vi "Main.Resize.vi"(10 "Sub Panel":refnum<vi>, 11 "VI in":refnum<vi>) -> ()   [LabVIEW 2019]
uses:
  <vilib>/Utility/miscctls.llb/LVPointTypeDef.ctl
  Users/Nicole/Downloads/a/ims-desktop/Variaveis/WindowAppearance.vi
  Users/Nicole/Downloads/a/ims-desktop/Variaveis/Config.vi
  Users/Nicole/Downloads/a/ims-desktop/Variaveis/Cnc.vi
  Users/Nicole/Downloads/a/ims-desktop/Variaveis/Checklist.vi
  Users/Nicole/Downloads/a/ims-desktop/Variaveis/NetworkShortcutLink.vi
  Users/Nicole/Downloads/a/ims-desktop/Variaveis/ProductionOrderConfiguration.vi
  Users/Nicole/Downloads/a/ims-desktop/Variaveis/CharacteristicVisualization.vi
  Users/Nicole/Downloads/a/ims-desktop/Variaveis/AnalogDigitalIOs.vi
panel:
  out "SFMVisible":bool
  out "ENSVisible":bool
  out "Position":dbl
  out "SubPnlTop":i32
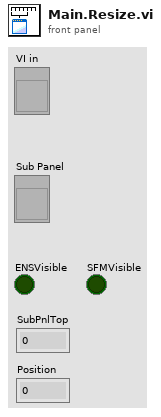
[diagram p1: front panel]
types:
  T1 = enum32{"Invalid", "Standard", "Closed", "Hidden", "Minimized", "Maximized"}
  T2 = typedef "LVPointTypeDef.ctl" = cluster{"Horizontal":i16, "Vertical":i16}
  T3 = typedef "LVAllMonitorsDisplayTypeDef.ctl" = cluster{"Bounds":cluster{"Left":i16, "Top":i16, "Right":i16, "Bottom":i16}, "Depth":i16}[]
  T4 = cluster{"Bounds":cluster{"Left":i16, "Top":i16, "Right":i16, "Bottom":i16}, "Depth":i16}
  T5 = cluster{"Left":i16, "Top":i16, "Right":i16, "Bottom":i16}
  T6 = cluster{"EnsPanelCode":i32, "GcfWorkcenterId":i32, "MeasurementType":i32, "SmartkattTemporaryFolder":path, "SmartkattReelFolder":path, "SmartkattConfiguration":string[][], "PrintReelLabel":bool, "Wire.TimeToCheckStatus":i32, "Wire.SegmentLength":i32, "EnablePopupAfterReelCut":bool}
  T7 = typedef "Msm.Checklist.ctl" = cluster{"checklistId":string, "plantId":i32, "departmentId":i32, "title":string, "version":i32, "createDate":timestamp, "userCreate":string, "language":string, "enabled":bool, "lists":cluster{"sequence":i32, "title":string, "description":string, "items":cluster{"sequence":i32, "title":string, "description":string, "type":enum16{"quantitative", "qualitative", "descriptive", "formula", "ensFindValue", "ensCharacteristic"}, "linearPosition":dbl, "angularPosition":dbl, "nominalValue":dbl, "minimumValue":dbl, "maximumValue":dbl, "unitOfMeasurement":string, "formula":string, "characteristic":string, "equipmentType":i32, "allowToleranceEdit":bool, "equipmentConfiguration":string}[]}[]}
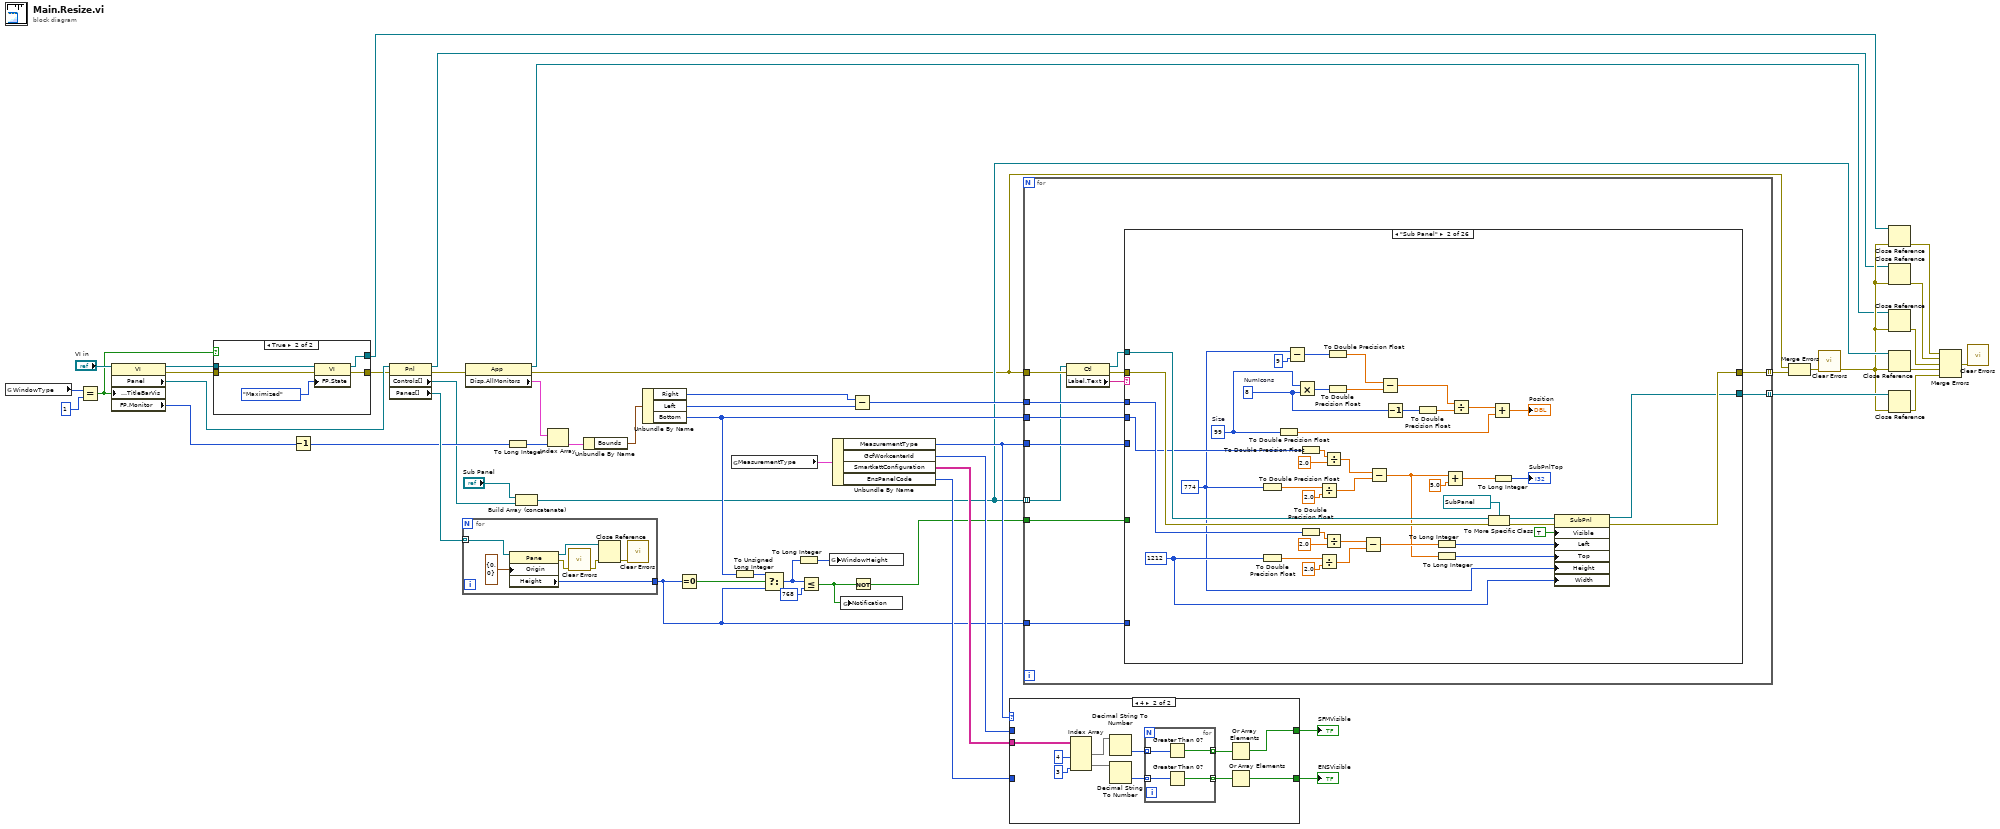
[diagram p0: block diagram]
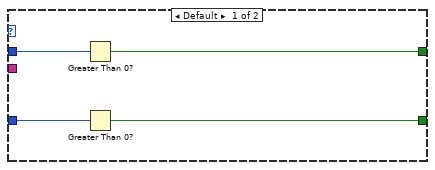
[diagram p3: hidden frame]
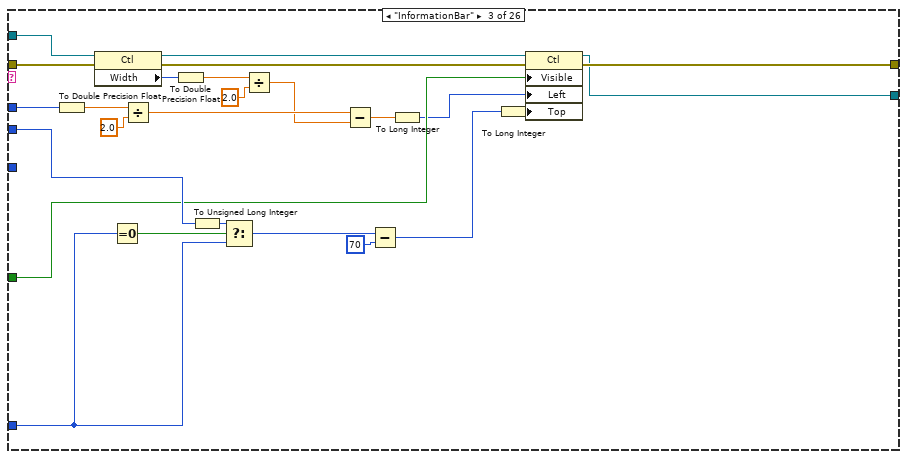
[diagram p5: hidden frame]
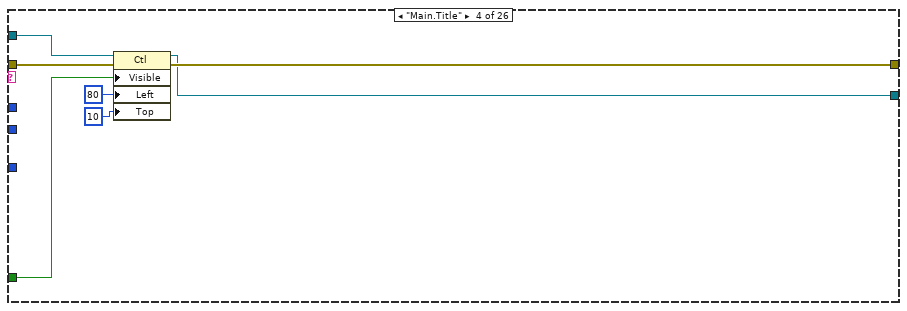
[diagram p6: hidden frame]
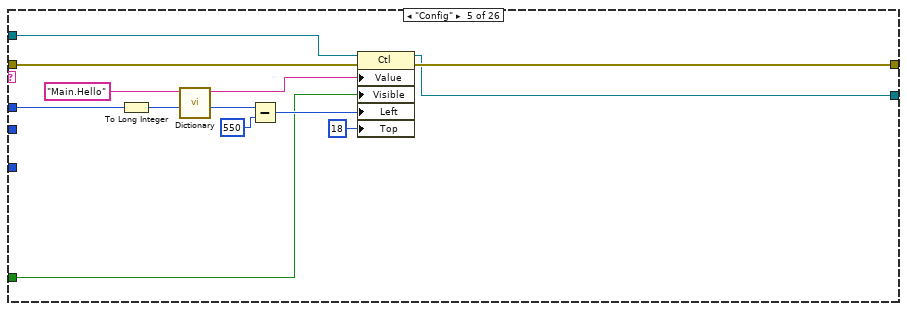
[diagram p7: hidden frame]
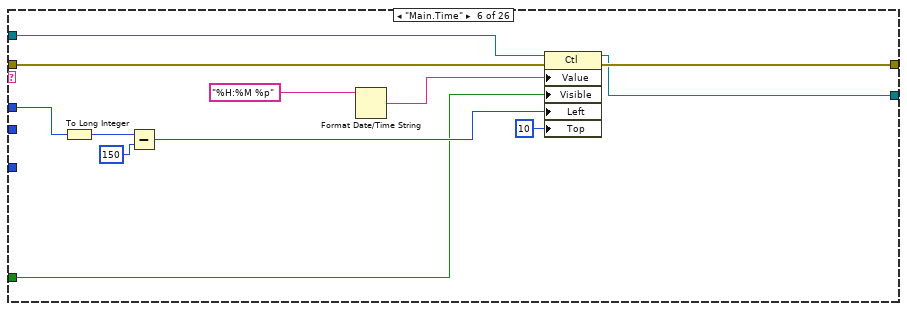
[diagram p8: hidden frame]
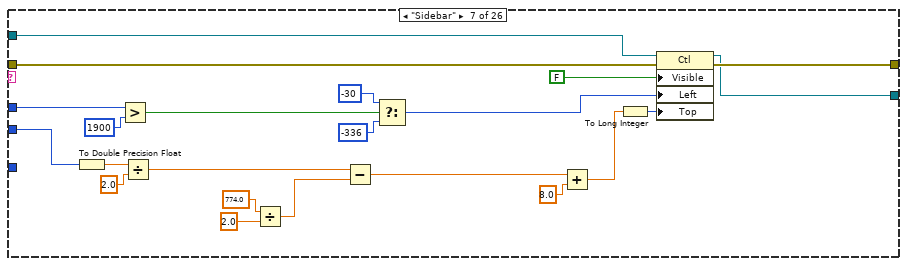
[diagram p9: hidden frame]
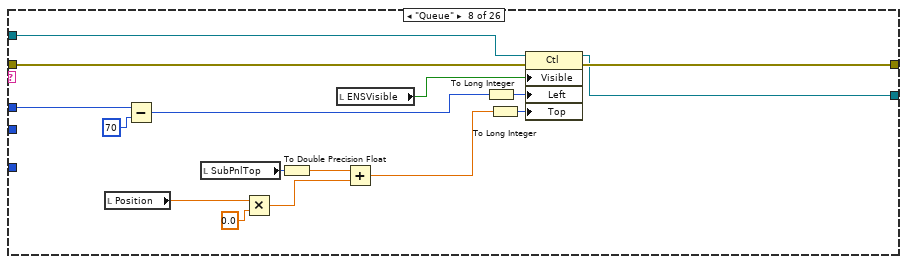
[diagram p10: hidden frame]
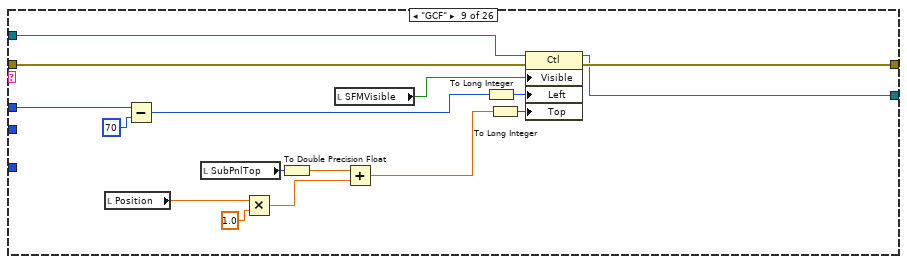
[diagram p11: hidden frame]
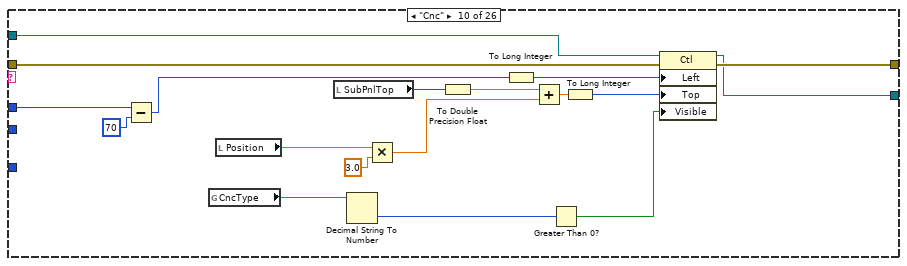
[diagram p12: hidden frame]
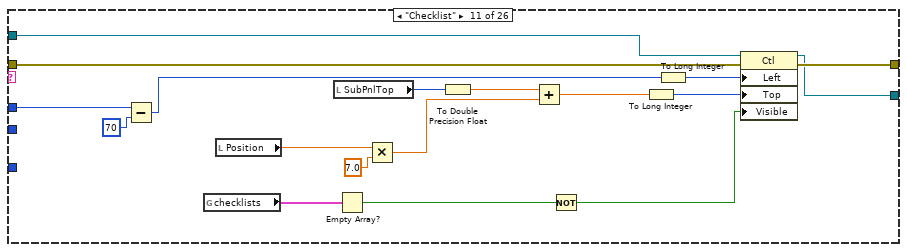
[diagram p13: hidden frame]
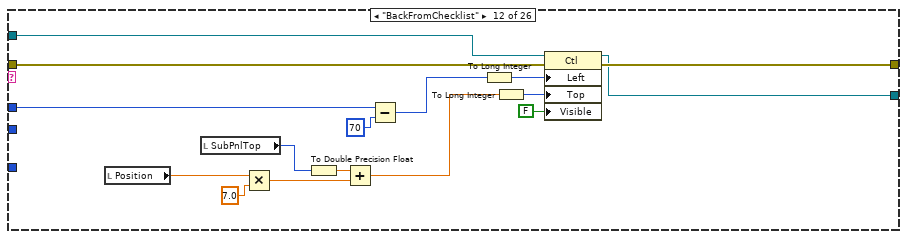
[diagram p14: hidden frame]
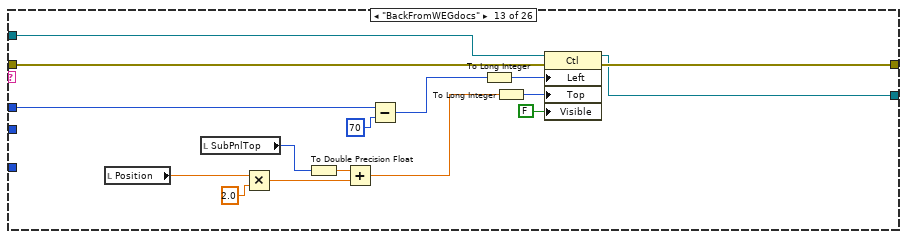
[diagram p15: hidden frame]
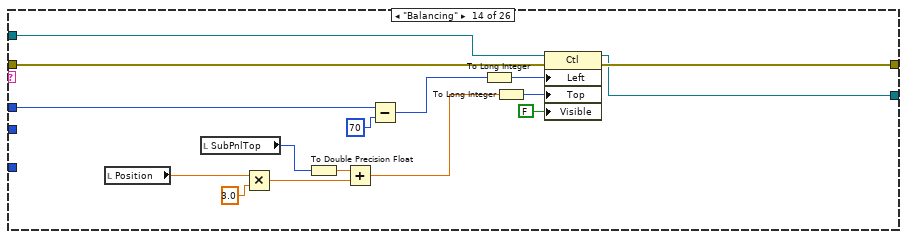
[diagram p16: hidden frame]
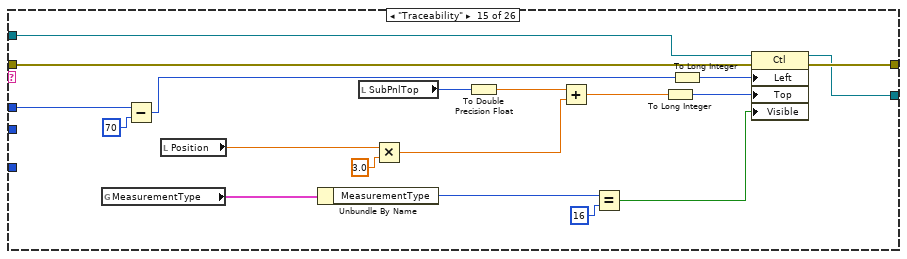
[diagram p17: hidden frame]
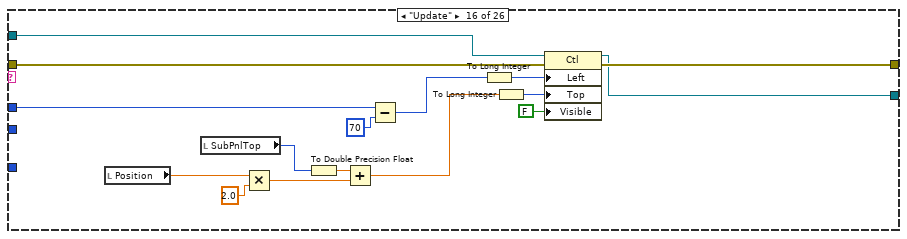
[diagram p18: hidden frame]
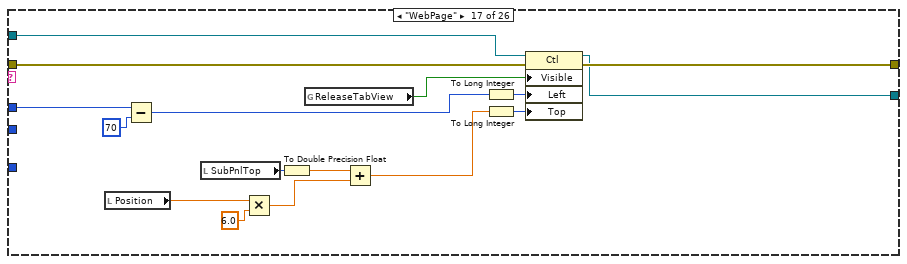
[diagram p19: hidden frame]
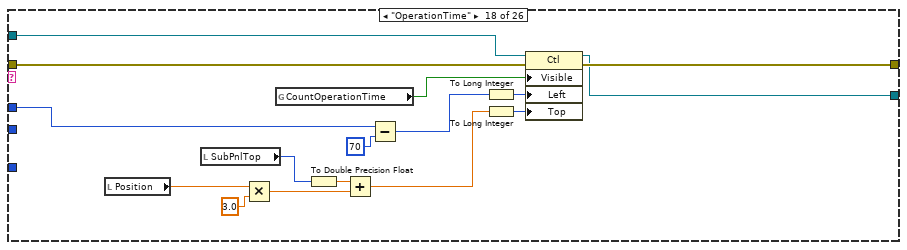
[diagram p20: hidden frame]
diagram:
  n1 = global read "WindowAppearance.vi" "WindowType"() -> (w39:i32)
  n2 = Equal?(x=w39, y=1) -> (x = y?=w18:bool)
  n3 = property class="VI"(reference="VI in", "Front Panel.TitleBarVis"=w18) -> (reference out=w19:refnum<vi>, error out=w21:errorcluster, "Panel"=w51:refnum<vi>, "FP.Monitor"=w46:u16)  [unwired: 1 in]
  n4 = case shown="True" w18 {
    tunnel: w21 -> [w54 w57]
    tunnel: [w54 w56] -> w20
    tunnel: w19 -> [w53 w58]
    tunnel: [w53 w55] -> w1
    frame False {
    }
    frame True {
      n5 = property class="VI"(reference=w58, error in=w57, "FP.State"=T1."Maximized" ("Front Panel Window:State")) -> (reference out=w55:refnum<vi>, error out=w56:errorcluster)
    }
  }
  n6 = Decrement(x=w46) -> (x-1=w43:u16)
  n7 = property class="Pnl"(reference=w51, error in=w20) -> (reference out=w2:refnum<vi>, error out=w29:errorcluster, "Controls[]"=w23:refnum<vi>[], "Panes[]"=w52:refnum<vi>[])
  n8 = for {
    tunnel: w52 -> [w66] mode=indexing
    tunnel: [w62] -> w28
    n9 = property class="Pane"(reference=w66, "Origin"=T2 {"Horizontal"=0, "Vertical"=0}) -> (reference out=w64:refnum<vi>, error out=w61:errorcluster, "Height"=w62:u32)  [unwired: 1 in]
    n10 = call <vilib>:"Clear Errors.vi"("error in (no error)"=w61) -> ("error out"=w60:errorcluster)  [unwired: 5 in, 1 out]
    n11 = Close Reference(reference=w64, error in (no error)=w60) -> (error out=w63:errorcluster)
    n12 = call <vilib>:"Clear Errors.vi"("error in (no error)"=w63) -> ()  [unwired: 5 in, 2 out]
  }
  n13 = property class="App"(error in=w29) -> (reference out=w3:refnum<vi>, error out=w8:errorcluster, "Disp.AllMonitors"=w47:T3)  [unwired: 1 in]
  n14 = To Long Integer(number=w43) -> (32bit integer=w17:i32)
  n15 = Build Array (concatenate)("Sub Panel", w23) -> (w14:refnum<vi>[])
  n16 = Index Array(array=w47, index=w17) -> (element=w45:T4)
  n17 = Unbundle By Name(w45) -> ("Bounds"=w44:T5)
  n18 = Unbundle By Name(w44) -> ("Right"=w42:i16, "Left"=w41:i16, "Bottom"=w36:i16)
  n19 = Equal To 0?(x=w28) -> (x = 0?=w37:bool)
  n20 = global read "Config.vi" "MeasurementType"() -> (w48:T6)
  n21 = To Unsigned Long Integer(number=w36) -> (unsigned 32bit integer=w16:u32)
  n22 = Select(t=w16, s=w37, f=w28) -> (s? t:f=w35:u32)
  n23 = To Long Integer(number=w35) -> (32bit integer=w15:i32)
  n24 = Less Or Equal?(x=w35, y=u32 768) -> (x <= y?=w33:bool)
  n25 = global write "WindowAppearance.vi" "WindowHeight"(w15) -> ()
  n26 = Unbundle By Name(w48) -> ("MeasurementType"=w30:i32, "GcfWorkcenterId"=w49:i32, "SmartkattConfiguration"=w50:string[][], "EnsPanelCode"=w32:i32)
  n27 = global write "WindowAppearance.vi" "Notification"(w33) -> ()
  n28 = Subtract(x=w42, y=w41) -> (x-y=w40:i16)
  n29 = Not(x=w33) -> (.not. x?=w27:bool)
  n30 = case shown="4" w30 {
    tunnel: [w69 w76] -> w24
    tunnel: w49 -> [w70 _]
    tunnel: w50 -> [_ w81]
    tunnel: w32 -> [w68 _]
    tunnel: [w67 w71] -> w31
    frame Default {
      n31 = Greater Than 0?(x=w70) -> (x > 0?=w69:bool)
      n32 = Greater Than 0?(x=w68) -> (x > 0?=w67:bool)
    }
    frame 4 {
      n33 = Index Array(array=w81, index (col) #1=4 ("disabled index (col)"), index (col) #2=3 ("index (col)")) -> (element #1=w79:string[], element #2=w75:string[])  [unwired: 2 in]
      n34 = Decimal String To Number(string=w79) -> (number=w78:i32[])  [unwired: 2 in, 1 out]
      n35 = Decimal String To Number(string=w75) -> (number=w74:i32[])  [unwired: 2 in, 1 out]
      n36 = for {
        tunnel: w78 -> [w85] mode=indexing
        tunnel: [w84] -> w77 mode=indexing
        tunnel: w74 -> [w83] mode=indexing
        tunnel: [w82] -> w72 mode=indexing
        n37 = Greater Than 0?(x=w85) -> (x > 0?=w84:bool)
        n38 = Greater Than 0?(x=w83) -> (x > 0?=w82:bool)
      }
      n39 = Or Array Elements(Boolean array=w77) -> (logical OR=w76:bool)
      n40 = Or Array Elements(Boolean array=w72) -> (logical OR=w71:bool)
    }
  }
  "ENSVisible" <- w31
  "SFMVisible" <- w24
  n41 = for {
    tunnel: w40 -> [w97]
    tunnel: w36 -> [w96]
    tunnel: w28 -> [w94]
    tunnel: w30 -> [w93]
    tunnel: w14 -> [w87] mode=indexing
    tunnel: w27 -> [w92]
    tunnel: [w86] -> w12 mode=indexing
    tunnel: w8 -> [w88]
    tunnel: [w95] -> w26 mode=indexing
    n42 = property class="Ctl"(reference=w87, error in=w88) -> (reference out=w90:refnum<vi>, error out=w89:errorcluster, "Label.Text"=w91:string)
    n43 = case shown="\"Sub Panel\"" w91 {
      tunnel: w89 -> [w99 w140 w158 w171 w182 w196 w219 w236 w252 w270 w288 w304 w320 w336 w355 w371 w387 w403 w419 w439 w455 w475 w495 w511 w521 w531]
      tunnel: [w99 w137 w168 w175 w187 w199 w221 w237 w253 w271 w289 w305 w321 w337 w356 w372 w388 w404 w420 w440 w456 w476 w496 w512 w527 w533] -> w95
      tunnel: w90 -> [w98 w141 w160 w172 w181 w195 w218 w235 w251 w269 w287 w303 w319 w335 w354 w370 w386 w402 w418 w438 w454 w474 w494 w510 w523 w530]
      tunnel: w97 -> [_ w130 w162 _ w185 w194 w207 w234 w250 w268 w286 w302 w318 w334 w353 w369 w385 w401 w417 w437 w453 w473 w493 w509 w519 _]
      tunnel: w96 -> [_ w128 w153 _ _ _ w212 _ _ _ _ _ _ _ _ _ _ _ _ _ _ _ _ _ _ _]
      tunnel: w94 -> [_ _ w155 _ _ _ _ _ _ _ _ _ _ _ _ _ _ _ _ _ _ _ _ _ _ _]
      tunnel: w93 -> [_ _ _ _ _ _ _ _ _ _ _ _ _ _ _ _ _ _ _ w432 _ _ _ _ _ _]
      tunnel: w92 -> [_ _ w150 w170 w178 w190 _ _ _ _ _ _ _ _ _ _ _ _ _ _ _ _ _ _ _ _]
      tunnel: [w98 w110 w149 w169 w177 w189 w202 w225 w241 w257 w275 w293 w309 w325 w341 w360 w376 w392 w408 w424 w444 w460 w484 w500 w514 w528] -> w86
      frame Default {
      }
      frame "Sub Panel" {
        w113 = u32 99  # Size
        w112 = u32 8  # NumIcons
        w133 = u32 1212 ("Container Bounds:Width")
        w111 = u32 774 ("Container Bounds:Height")
        n44 = To Double Precision Float(number=w111) -> (double precision float=w103:dbl)
        n45 = To Double Precision Float(number=w133) -> (double precision float=w105:dbl)
        n46 = To Double Precision Float(number=w113) -> (double precision float=w101:dbl)
        n47 = Subtract(x=w111, y=u32 9) -> (x-y=w115:u32)
        n48 = Multiply(x=w113, y=w112) -> (x*y=w124:u32)
        n49 = To Double Precision Float(number=w128) -> (double precision float=w104:dbl)
        n50 = To Double Precision Float(number=w130) -> (double precision float=w106:dbl)
        n51 = Divide(x=w103, y=2.0) -> (x/y=w125:dbl)
        n52 = Divide(x=w105, y=2.0) -> (x/y=w132:dbl)
        n53 = Divide(x=w104, y=2.0) -> (x/y=w127:dbl)
        n54 = Divide(x=w106, y=2.0) -> (x/y=w135:dbl)
        n55 = To Double Precision Float(number=w115) -> (double precision float=w120:dbl)
        n56 = To Double Precision Float(number=w124) -> (double precision float=w102:dbl)
        n57 = Subtract(x=w135, y=w132) -> (x-y=w131:dbl)
        n58 = Subtract(x=w127, y=w125) -> (x-y=w119:dbl)
        n59 = Subtract(x=w120, y=w102) -> (x-y=w123:dbl)
        n60 = Decrement(x=w112) -> (x-1=w122:u32)
        n61 = To Double Precision Float(number=w122) -> (double precision float=w100:dbl)
        n62 = To Long Integer(number=w131) -> (32bit integer=w107:i32)
        n63 = To Long Integer(number=w119) -> (32bit integer=w108:i32)
        n64 = Add(x=w119, y=5.0) -> (x+y=w118:dbl)
        n65 = Divide(x=w123, y=w100) -> (x/y=w121:dbl)
        n66 = To More Specific Class(target class=refnum<vi> refnum ("reference"), reference=w141, error in=w140) -> (specific class reference=w138:refnum<vi>, error out=w139:errorcluster)
        n67 = Add(x=w121, y=w101) -> (x+y=→"Position":dbl)
        n68 = To Long Integer(number=w118) -> (32bit integer=→"SubPnlTop":i32)
        n69 = property class="SubPnl"(reference=w138, error in=w139, "Visible"=TRUE, "Left"=w107, "Top"=w108, "Height"=w111, "Width"=w133) -> (reference out=w110:refnum<vi>, error out=w137:errorcluster)
      }
      frame "InformationBar" {
        n70 = To Double Precision Float(number=w162) -> (double precision float=w144:dbl)
        n71 = property class="Ctl"(reference=w160, error in=w158) -> (reference out=w159:refnum<vi>, error out=w157:errorcluster, "Width"=w161:u32)
        n72 = Equal To 0?(x=w155) -> (x = 0?=w156:bool)
        n73 = Divide(x=w144, y=2.0) -> (x/y=w166:dbl)
        n74 = To Double Precision Float(number=w161) -> (double precision float=w145:dbl)
        n75 = To Unsigned Long Integer(number=w153) -> (unsigned 32bit integer=w148:u32)
        n76 = Select(t=w148, s=w156, f=w155) -> (s? t:f=w152:u32)
        n77 = Divide(x=w145, y=2.0) -> (x/y=w164:dbl)
        n78 = Subtract(x=w166, y=w164) -> (x-y=w163:dbl)
        n79 = Subtract(x=w152, y=u32 70) -> (x-y=w151:u32)
        n80 = To Long Integer(number=w163) -> (32bit integer=w147:i32)
        n81 = To Long Integer(number=w151) -> (32bit integer=w146:i32)
        n82 = property class="Ctl"(reference=w159, error in=w157, "Visible"=w150, "Left"=w147, "Top"=w146) -> (reference out=w149:refnum<vi>, error out=w168:errorcluster)
      }
      frame "Main.Title" {
        n83 = property class="Ctl"(reference=w172, error in=w171, "Visible"=w170, "Left"=80 ("Position:Left"), "Top"=10 ("Position:Top")) -> (reference out=w169:refnum<vi>, error out=w175:errorcluster)
      }
      frame "Config" {
        n84 = To Long Integer(number=w185) -> (32bit integer=w176:i32)
        n85 = call "Dictionary.vi"("String"="Main.Hello") -> ("Traducao"=w180:string)  [unwired: 10 in]
        n86 = Subtract(x=w176, y=550) -> (x-y=w183:i32)
        n87 = property class="Ctl"(reference=w181, error in=w182, "Value"=w180, "Visible"=w178, "Left"=w183, "Top"=18 ("Position:Top")) -> (reference out=w177:refnum<vi>, error out=w187:errorcluster)
      }
      frame "Main.Time" {
        n88 = To Long Integer(number=w194) -> (32bit integer=w188:i32)
        n89 = Subtract(x=w188, y=150) -> (x-y=w192:i32)
        n90 = Format Date/Time String(time format string (%c)="%H:%M %p") -> (date/time string=w197:string)  [unwired: 2 in]
        n91 = property class="Ctl"(reference=w195, error in=w196, "Value"=w197, "Visible"=w190, "Left"=w192, "Top"=10 ("Position:Top")) -> (reference out=w189:refnum<vi>, error out=w199:errorcluster)
      }
      frame "Sidebar" {
        n92 = To Double Precision Float(number=w212) -> (double precision float=w201:dbl)
        n93 = Greater?(x=w207, y=i16 1900) -> (0:w206:bool)
        n94 = Divide(x=w201, y=2.0) -> (x/y=w216:dbl)
        n95 = Divide(x=774.0 ("Container Bounds:Height"), y=2.0) -> (x/y=w217:dbl)
        n96 = Subtract(x=w216, y=w217) -> (x-y=w211:dbl)
        n97 = Select(t=-30 ("Position:Left"), s=w206, f=-336 ("Position:Left")) -> (s? t:f=w203:i32)
        n98 = Add(x=w211, y=8.0) -> (x+y=w210:dbl)
        n99 = To Long Integer(number=w210) -> (32bit integer=w200:i32)
        n100 = property class="Ctl"(reference=w218, error in=w219, "Visible"=FALSE, "Left"=w203, "Top"=w200) -> (reference out=w202:refnum<vi>, error out=w221:errorcluster)
      }
      frame "Queue" {
        n101 = local read "Position"() -> (w231:dbl)
        n102 = Subtract(x=w234, y=i16 70) -> (x-y=w232:i16)
        n103 = local read "SubPnlTop"() -> (w228:i32)
        n104 = Multiply(x=w231, y=0.0) -> (x*y=w229:dbl)
        n105 = To Double Precision Float(number=w228) -> (double precision float=w224:dbl)
        n106 = local read "ENSVisible"() -> (w226:bool)
        n107 = Add(x=w224, y=w229) -> (x+y=w227:dbl)
        n108 = To Long Integer(number=w232) -> (32bit integer=w223:i32)
        n109 = To Long Integer(number=w227) -> (32bit integer=w222:i32)
        n110 = property class="Ctl"(reference=w235, error in=w236, "Visible"=w226, "Left"=w223, "Top"=w222) -> (reference out=w225:refnum<vi>, error out=w237:errorcluster)
      }
      frame "GCF" {
        n111 = local read "Position"() -> (w247:dbl)
        n112 = Subtract(x=w250, y=i16 70) -> (x-y=w248:i16)
        n113 = local read "SubPnlTop"() -> (w245:i32)
        n114 = Multiply(x=w247, y=1.0) -> (x*y=w246:dbl)
        n115 = To Double Precision Float(number=w245) -> (double precision float=w238:dbl)
        n116 = local read "SFMVisible"() -> (w242:bool)
        n117 = Add(x=w238, y=w246) -> (x+y=w243:dbl)
        n118 = To Long Integer(number=w248) -> (32bit integer=w240:i32)
        n119 = To Long Integer(number=w243) -> (32bit integer=w239:i32)
        n120 = property class="Ctl"(reference=w251, error in=w252, "Visible"=w242, "Left"=w240, "Top"=w239) -> (reference out=w241:refnum<vi>, error out=w253:errorcluster)
      }
      frame "Cnc" {
        n121 = Subtract(x=w268, y=i16 70) -> (x-y=w266:i16)
        n122 = global read "Cnc.vi" "CncType"() -> (w264:string)
        n123 = local read "Position"() -> (w263:dbl)
        n124 = local read "SubPnlTop"() -> (w261:i32)
        n125 = Decimal String To Number(string=w264) -> (number=w265:i32)  [unwired: 2 in, 1 out]
        n126 = Multiply(x=w263, y=3.0) -> (x*y=w262:dbl)
        n127 = To Double Precision Float(number=w261) -> (double precision float=w256:dbl)
        n128 = To Long Integer(number=w266) -> (32bit integer=w255:i32)
        n129 = Add(x=w256, y=w262) -> (x+y=w259:dbl)
        n130 = Greater Than 0?(x=w265) -> (x > 0?=w258:bool)
        n131 = To Long Integer(number=w259) -> (32bit integer=w254:i32)
        n132 = property class="Ctl"(reference=w269, error in=w270, "Left"=w255, "Top"=w254, "Visible"=w258) -> (reference out=w257:refnum<vi>, error out=w271:errorcluster)
      }
      frame "Checklist" {
        n133 = Subtract(x=w286, y=i16 70) -> (x-y=w284:i16)
        n134 = global read "Checklist.vi" "checklists"() -> (w278:T7[])
        n135 = local read "Position"() -> (w283:dbl)
        n136 = local read "SubPnlTop"() -> (w281:i32)
        n137 = Empty Array?(array=w278) -> (empty?=w277:bool)
        n138 = Multiply(x=w283, y=7.0) -> (x*y=w282:dbl)
        n139 = To Double Precision Float(number=w281) -> (double precision float=w274:dbl)
        n140 = Add(x=w274, y=w282) -> (x+y=w279:dbl)
        n141 = Not(x=w277) -> (.not. x?=w276:bool)
        n142 = To Long Integer(number=w279) -> (32bit integer=w272:i32)
        n143 = To Long Integer(number=w284) -> (32bit integer=w273:i32)
        n144 = property class="Ctl"(reference=w287, error in=w288, "Left"=w273, "Top"=w272, "Visible"=w276) -> (reference out=w275:refnum<vi>, error out=w289:errorcluster)
      }
      frame "BackFromChecklist" {
        n145 = local read "Position"() -> (w299:dbl)
        n146 = local read "SubPnlTop"() -> (w297:i32)
        n147 = Multiply(x=w299, y=7.0) -> (x*y=w298:dbl)
        n148 = To Double Precision Float(number=w297) -> (double precision float=w290:dbl)
        n149 = Add(x=w290, y=w298) -> (x+y=w295:dbl)
        n150 = Subtract(x=w302, y=i16 70) -> (x-y=w300:i16)
        n151 = To Long Integer(number=w300) -> (32bit integer=w292:i32)
        n152 = To Long Integer(number=w295) -> (32bit integer=w291:i32)
        n153 = property class="Ctl"(reference=w303, error in=w304, "Left"=w292, "Top"=w291, "Visible"=FALSE) -> (reference out=w293:refnum<vi>, error out=w305:errorcluster)
      }
      frame "BackFromWEGdocs" {
        n154 = local read "Position"() -> (w315:dbl)
        n155 = local read "SubPnlTop"() -> (w313:i32)
        n156 = Multiply(x=w315, y=2.0) -> (x*y=w314:dbl)
        n157 = To Double Precision Float(number=w313) -> (double precision float=w308:dbl)
        n158 = Add(x=w308, y=w314) -> (x+y=w311:dbl)
        n159 = Subtract(x=w318, y=i16 70) -> (x-y=w316:i16)
        n160 = To Long Integer(number=w316) -> (32bit integer=w307:i32)
        n161 = To Long Integer(number=w311) -> (32bit integer=w306:i32)
        n162 = property class="Ctl"(reference=w319, error in=w320, "Left"=w307, "Top"=w306, "Visible"=FALSE) -> (reference out=w309:refnum<vi>, error out=w321:errorcluster)
      }
      frame "Balancing" {
        n163 = local read "Position"() -> (w330:dbl)
        n164 = local read "SubPnlTop"() -> (w328:i32)
        n165 = Multiply(x=w330, y=3.0) -> (x*y=w329:dbl)
        n166 = To Double Precision Float(number=w328) -> (double precision float=w322:dbl)
        n167 = Add(x=w322, y=w329) -> (x+y=w326:dbl)
        n168 = Subtract(x=w334, y=i16 70) -> (x-y=w332:i16)
        n169 = To Long Integer(number=w332) -> (32bit integer=w324:i32)
        n170 = To Long Integer(number=w326) -> (32bit integer=w323:i32)
        n171 = property class="Ctl"(reference=w335, error in=w336, "Left"=w324, "Top"=w323, "Visible"=FALSE) -> (reference out=w325:refnum<vi>, error out=w337:errorcluster)
      }
      frame "Traceability" {
        n172 = global read "Config.vi" "MeasurementType"() -> (w349:T6)
        n173 = Subtract(x=w353, y=i16 70) -> (x-y=w351:i16)
        n174 = local read "Position"() -> (w347:dbl)
        n175 = Unbundle By Name(w349) -> ("MeasurementType"=w350:i32)
        n176 = local read "SubPnlTop"() -> (w345:i32)
        n177 = Multiply(x=w347, y=3.0) -> (x*y=w346:dbl)
        n178 = To Double Precision Float(number=w345) -> (double precision float=w338:dbl)
        n179 = Add(x=w338, y=w346) -> (x+y=w343:dbl)
        n180 = Equal?(x=w350, y=16) -> (x = y?=w342:bool)
        n181 = To Long Integer(number=w343) -> (32bit integer=w339:i32)
        n182 = To Long Integer(number=w351) -> (32bit integer=w340:i32)
        n183 = property class="Ctl"(reference=w354, error in=w355, "Left"=w340, "Top"=w339, "Visible"=w342) -> (reference out=w341:refnum<vi>, error out=w356:errorcluster)
      }
      frame "Update" {
        n184 = local read "Position"() -> (w365:dbl)
        n185 = local read "SubPnlTop"() -> (w363:i32)
        n186 = Multiply(x=w365, y=2.0) -> (x*y=w364:dbl)
        n187 = To Double Precision Float(number=w363) -> (double precision float=w357:dbl)
        n188 = Add(x=w357, y=w364) -> (x+y=w361:dbl)
        n189 = Subtract(x=w369, y=i16 70) -> (x-y=w367:i16)
        n190 = To Long Integer(number=w367) -> (32bit integer=w359:i32)
        n191 = To Long Integer(number=w361) -> (32bit integer=w358:i32)
        n192 = property class="Ctl"(reference=w370, error in=w371, "Left"=w359, "Top"=w358, "Visible"=FALSE) -> (reference out=w360:refnum<vi>, error out=w372:errorcluster)
      }
      frame "WebPage" {
        n193 = local read "Position"() -> (w381:dbl)
        n194 = Subtract(x=w385, y=i16 70) -> (x-y=w383:i16)
        n195 = local read "SubPnlTop"() -> (w379:i32)
        n196 = Multiply(x=w381, y=6.0) -> (x*y=w380:dbl)
        n197 = To Double Precision Float(number=w379) -> (double precision float=w375:dbl)
        n198 = global read "NetworkShortcutLink.vi" "ReleaseTabView"() -> (w382:bool)
        n199 = Add(x=w375, y=w380) -> (x+y=w377:dbl)
        n200 = To Long Integer(number=w383) -> (32bit integer=w374:i32)
        n201 = To Long Integer(number=w377) -> (32bit integer=w373:i32)
        n202 = property class="Ctl"(reference=w386, error in=w387, "Visible"=w382, "Left"=w374, "Top"=w373) -> (reference out=w376:refnum<vi>, error out=w388:errorcluster)
      }
      frame "OperationTime" {
        n203 = local read "Position"() -> (w398:dbl)
        n204 = local read "SubPnlTop"() -> (w396:i32)
        n205 = Multiply(x=w398, y=3.0) -> (x*y=w397:dbl)
        n206 = global read "ProductionOrderConfiguration.vi" "CountOperationTime"() -> (w393:bool)
        n207 = To Double Precision Float(number=w396) -> (double precision float=w389:dbl)
        n208 = Add(x=w389, y=w397) -> (x+y=w394:dbl)
        n209 = Subtract(x=w401, y=i16 70) -> (x-y=w399:i16)
        n210 = To Long Integer(number=w399) -> (32bit integer=w391:i32)
        n211 = To Long Integer(number=w394) -> (32bit integer=w390:i32)
        n212 = property class="Ctl"(reference=w402, error in=w403, "Visible"=w393, "Left"=w391, "Top"=w390) -> (reference out=w392:refnum<vi>, error out=w404:errorcluster)
      }
      frame "VirtualKeyboard" {
        n213 = Subtract(x=w417, y=i16 70) -> (x-y=w415:i16)
        n214 = local read "Position"() -> (w413:dbl)
        n215 = local read "SubPnlTop"() -> (w411:i32)
        n216 = Multiply(x=w413, y=4.0) -> (x*y=w412:dbl)
        n217 = To Long Integer(number=w415) -> (32bit integer=w405:i32)
        n218 = To Double Precision Float(number=w411) -> (double precision float=w407:dbl)
        n219 = global read "WindowAppearance.vi" "ShowVirtualKeyboardButton"() -> (w414:bool)
        n220 = Add(x=w407, y=w412) -> (x+y=w409:dbl)
        n221 = To Long Integer(number=w409) -> (32bit integer=w406:i32)
        n222 = property class="Ctl"(reference=w418, error in=w419, "Visible"=w414, "Left"=w405, "Top"=w406) -> (reference out=w408:refnum<vi>, error out=w420:errorcluster)
      }
      frame "QGA" {
        n223 = Not Equal?(x=w432, y=11) -> (x != y?=w431:bool)
        n224 = local read "Position"() -> (w429:dbl)
        n225 = Subtract(x=w437, y=i16 70) -> (x-y=w435:i16)
        n226 = global read "CharacteristicVisualization.vi" "EnableCharacteristicVisualization"() -> (w434:bool)
        n227 = Multiply(x=w429, y=5.0) -> (x*y=w428:dbl)
        n228 = local read "SubPnlTop"() -> (w427:i32)
        n229 = To Double Precision Float(number=w427) -> (double precision float=w421:dbl)
        n230 = Add(x=w421, y=w428) -> (x+y=w425:dbl)
        n231 = And(x=w434, y=w431) -> (x .and. y?=w433:bool)
        n232 = To Long Integer(number=w425) -> (32bit integer=w422:i32)
        n233 = To Long Integer(number=w435) -> (32bit integer=w423:i32)
        n234 = property class="Ctl"(reference=w438, error in=w439, "Visible"=w433, "Left"=w423, "Top"=w422) -> (reference out=w424:refnum<vi>, error out=w440:errorcluster)
      }
      frame "Back" {
        n235 = local read "Position"() -> (w450:dbl)
        n236 = local read "SubPnlTop"() -> (w448:i32)
        n237 = Multiply(x=w450, y=5.0) -> (x*y=w449:dbl)
        n238 = To Double Precision Float(number=w448) -> (double precision float=w441:dbl)
        n239 = Add(x=w441, y=w449) -> (x+y=w446:dbl)
        n240 = Subtract(x=w453, y=i16 70) -> (x-y=w451:i16)
        n241 = To Long Integer(number=w446) -> (32bit integer=w442:i32)
        n242 = To Long Integer(number=w451) -> (32bit integer=w443:i32)
        n243 = property class="Ctl"(reference=w454, error in=w455, "Visible"=FALSE, "Left"=w443, "Top"=w442) -> (reference out=w444:refnum<vi>, error out=w456:errorcluster)
      }
      frame "TemperatureHumidity" {
        n244 = global read "AnalogDigitalIOs.vi" "AnalogDigitalIO"() -> (w465:string[][])
        n245 = Index Array(array=w465, index (col)=3 ("disabled index (col)")) -> (element=w464:string[])  [unwired: 1 in]
        n246 = for {
          tunnel: w464 -> [w478] mode=indexing
          tunnel: [w477] -> w461 mode=indexing
          n247 = case shown="Default" w478 {
            tunnel: [TRUE FALSE] -> w477
            frame "70", "71", "72", "73", "74", "75", "76", "77", "80" {
            }
            frame Default {
            }
          }
        }
        n248 = Subtract(x=w473, y=i16 70) -> (x-y=w471:i16)
        n249 = To Long Integer(number=w471) -> (32bit integer=w458:i32)
        n250 = local read "Position"() -> (w470:dbl)
        n251 = local read "SubPnlTop"() -> (w468:i32)
        n252 = Multiply(x=w470, y=7.0) -> (x*y=w469:dbl)
        n253 = To Double Precision Float(number=w468) -> (double precision float=w457:dbl)
        n254 = Or Array Elements(Boolean array=w461) -> (logical OR=w462:bool)
        n255 = Add(x=w457, y=w469) -> (x+y=w466:dbl)
        n256 = To Long Integer(number=w466) -> (32bit integer=w459:i32)
        n257 = property class="Ctl"(reference=w474, error in=w475, "Visible"=w462, "Left"=w458, "Top"=w459) -> (reference out=w460:refnum<vi>, error out=w476:errorcluster)
      }
      frame "Lunch" {
        n258 = local read "Position"() -> (w489:dbl)
        n259 = local read "SubPnlTop"() -> (w487:i32)
        n260 = Multiply(x=w489, y=6.0) -> (x*y=w488:dbl)
        n261 = To Double Precision Float(number=w487) -> (double precision float=w481:dbl)
        n262 = Add(x=w481, y=w488) -> (x+y=w485:dbl)
        n263 = Subtract(x=w493, y=i16 70) -> (x-y=w491:i16)
        n264 = To Long Integer(number=w485) -> (32bit integer=w482:i32)
        n265 = To Long Integer(number=w491) -> (32bit integer=w483:i32)
        n266 = property class="Ctl"(reference=w494, error in=w495, "Visible"=FALSE, "Left"=w483, "Top"=w482) -> (reference out=w484:refnum<vi>, error out=w496:errorcluster)
      }
      frame "WEGdoc" {
        n267 = local read "Position"() -> (w506:dbl)
        n268 = local read "SubPnlTop"() -> (w504:i32)
        n269 = Multiply(x=w506, y=2.0) -> (x*y=w505:dbl)
        n270 = To Double Precision Float(number=w504) -> (double precision float=w499:dbl)
        n271 = Add(x=w499, y=w505) -> (x+y=w502:dbl)
        n272 = Subtract(x=w509, y=i16 70) -> (x-y=w507:i16)
        n273 = To Long Integer(number=w502) -> (32bit integer=w497:i32)
        n274 = To Long Integer(number=w507) -> (32bit integer=w498:i32)
        n275 = property class="Ctl"(reference=w510, error in=w511, "Visible"=TRUE, "Left"=w498, "Top"=w497) -> (reference out=w500:refnum<vi>, error out=w512:errorcluster)
      }
      frame "OperationTimeSlider" {
        n276 = Increment(x=w519) -> (x+1=w518:i16)
        n277 = global read "ProductionOrderConfiguration.vi" "CountOperationTime"() -> (w515:bool)
        n278 = To More Specific Class(target class=refnum<vi> refnum ("OperationTimeSlider"), reference=w523, error in=w521) -> (specific class reference=w522:refnum<vi>, error out=w520:errorcluster)
        n279 = To Unsigned Long Integer(number=w518) -> (unsigned 32bit integer=w513:u32)
        n280 = property class="Slide (strict)"(reference=w522, error in=w520, "Visible"=w515, "Left"=-2 ("Position:Left"), "Top"=-1 ("Position:Top"), "Width"=w513, "Fill Color"=u32 38400, "Value"=0.0) -> (reference out=w514:refnum<vi>, error out=w527:errorcluster)
      }
      frame "WEGLogo.Picture" {
        w529 = 0 ("Position:Left")
        n281 = property class="Ctl"(reference=w530, error in=w531, "Visible"=TRUE, "Left"=w529, "Top"=w529) -> (reference out=w528:refnum<vi>, error out=w533:errorcluster)
      }
    }
  }
  n282 = Merge Errors(w8, w26) -> (w9:errorcluster)
  n283 = call <vilib>:"Clear Errors.vi"("error in (no error)"=w9) -> ("error out"=w7:errorcluster)  [unwired: 5 in, 1 out]
  n284 = Close Reference(reference=w1, error in (no error)=w7) -> (error out=w4:errorcluster)
  n285 = Close Reference(reference=w2, error in (no error)=w7) -> (error out=w5:errorcluster)
  n286 = Close Reference(reference=w3, error in (no error)=w7) -> (error out=w6:errorcluster)
  n287 = Close Reference(reference=w14, error in (no error)=w7) -> (error out=w13:errorcluster)
  n288 = Close Reference(reference=w12, error in (no error)=w7) -> (error out=w10:errorcluster)
  n289 = Merge Errors(w4, w5, w6, w13, w10) -> (w11:errorcluster)
  n290 = call <vilib>:"Clear Errors.vi"("error in (no error)"=w11) -> ()  [unwired: 5 in, 2 out]
